vi "HumanActionCache.vi"(6 "State":i32, 8 "Right X":dbl, 9 "Right Y":dbl, 10 "Left X":dbl, 11 "Left Y":dbl) -> (2 "RightMotorDemand":dbl, 3 "LeftMotorDemand":dbl)   [LabVIEW 2020]
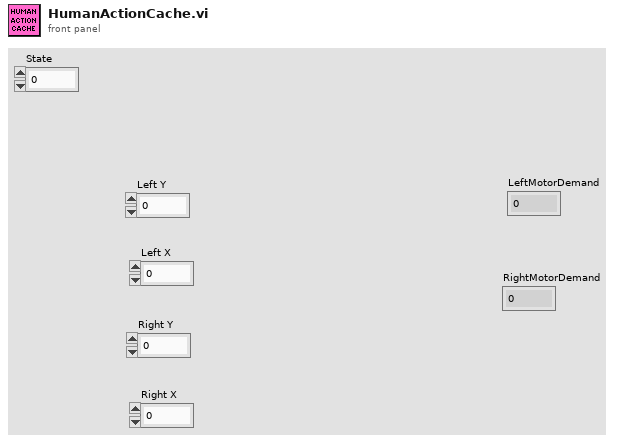
[diagram p1: front panel]
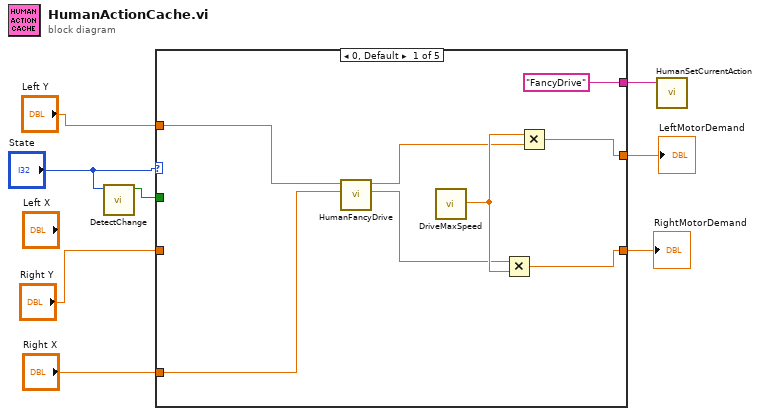
[diagram p0: block diagram]
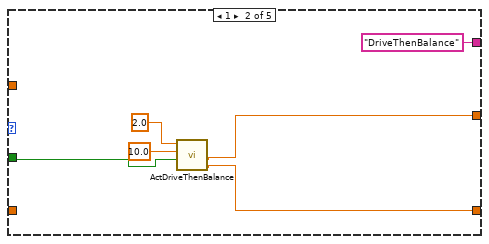
[diagram p2: hidden frame]
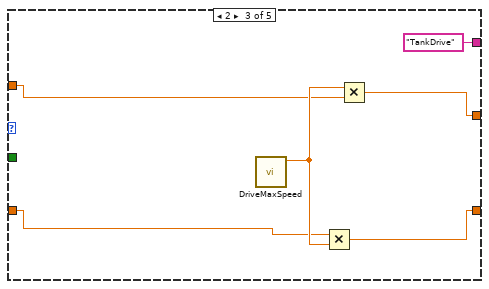
[diagram p3: hidden frame]
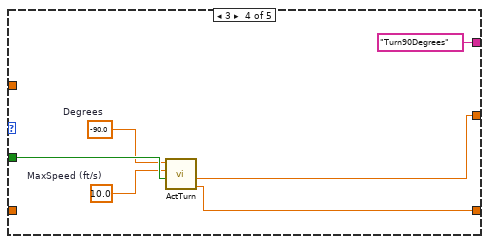
[diagram p4: hidden frame]
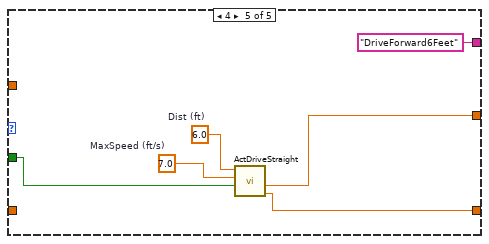
[diagram p5: hidden frame]
diagram:
  n1 = call "DetectChange.vi"("Value"="State") -> ("Changed"=w2:bool)  [unwired: 10 in]
  n2 = case shown="0, Default" "State" {
    tunnel: "Left Y" -> [w11 _ w27 _ _]
    tunnel: "Right X" -> [w10 _ _ _ _]
    tunnel: [w14 w22 w24 w34 w37] -> w6
    tunnel: [w15 w21 w25 w33 w36] -> w5
    tunnel: "Right Y" -> [_ _ w26 _ _]
    tunnel: w2 -> [_ w18 _ w32 w40]
    tunnel: ["FancyDrive" "DriveThenBalance" "TankDrive" "Turn90Degrees" "DriveForward6Feet"] -> w1
    frame 0, Default {
      n3 = call "HumanFancyDrive.vi"("X Axis"=w10, "Y Axis"=w11) -> ("Right Motor Value"=w12:dbl, "Left Motor Value"=w13:dbl)  [unwired: 8 in]
      n4 = call "DriveMaxSpeed.vi"() -> ("Max Speed (ft/sec)"=w16:dbl)  [unwired: 11 in]
      n5 = Multiply(x=w12, y=w16) -> (x*y=w15:dbl)
      n6 = Multiply(x=w16, y=w13) -> (x*y=w14:dbl)
    }
    frame 1 {
      n7 = call "ActDriveThenBalance.vi"("FirstTime"=w18, "MaxSpeed (ft/s)"=10.0, "Dist (ft)"=2.0) -> ("RightSpeedDemand"=w21:dbl, "LeftSpeedDemand"=w22:dbl)  [unwired: 6 in, 1 out]
    }
    frame 2 {
      n8 = call "DriveMaxSpeed.vi"() -> ("Max Speed (ft/sec)"=w28:dbl)  [unwired: 11 in]
      n9 = Multiply(x=w26, y=w28) -> (x*y=w25:dbl)
      n10 = Multiply(x=w28, y=w27) -> (x*y=w24:dbl)
    }
    frame 3 {
      w30 = -90.0  # Degrees
      w31 = 10.0  # MaxSpeed (ft/s)
      n11 = call "ActTurn.vi"("FirstTime"=w32, "MaxSpeed (ft/s)"=w31, "Degrees"=w30) -> ("RightSpeedDemand"=w33:dbl, "LeftSpeedDemand"=w34:dbl)  [unwired: 6 in, 1 out]
    }
    frame 4 {
      w38 = 7.0  # MaxSpeed (ft/s)
      w39 = 6.0  # Dist (ft)
      n12 = call "ActDriveStraight.vi"("FirstTime"=w40, "MaxSpeed (ft/s)"=w38, "Dist (ft)"=w39) -> ("RightSpeedDemand"=w36:dbl, "LeftSpeedDemand"=w37:dbl)  [unwired: 6 in, 1 out]
    }
  }
  "LeftMotorDemand" <- w6
  "RightMotorDemand" <- w5
  n13 = call "HumanSetCurrentAction.vi"("CurrentState"=w1) -> ()  [unwired: 11 in]
